vi "ITM10_test.vi"(7 "channel":i32=1, 11 "visa_in":refnum<visa-resource-name>="COM34") -> (0 "err_out":errorcluster={"status"=FALSE, "code"=1073676294, "source"="VISA Read in thcd_get_chan.vi"}, 2 "value":dbl, 4 "status":bool=TRUE, 5 "message":string)   [LabVIEW 2019]
panel:
  out "response V":string
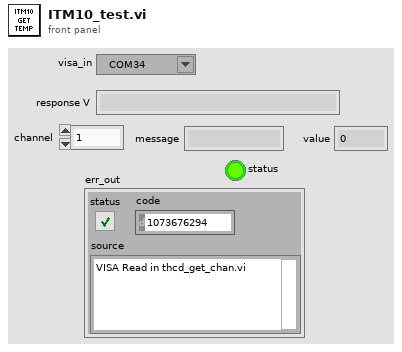
[diagram p1: front panel]
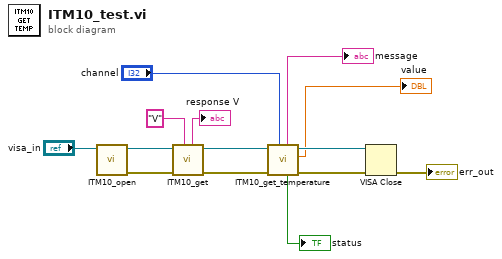
[diagram p0: block diagram]
diagram:
  n1 = call "ITM10_open.vi"("VISA in"="visa_in") -> ("error out"=w3:errorcluster, "VISA out"=w2:refnum<visa-resource-name>)  [unwired: 9 in]
  n2 = call "ITM10_get.vi"("command"="V", "error in"=w3, "VISA_ref_in"=w2) -> ("error out"=w10:errorcluster, "VISA_ref_out"=w11:refnum<visa-resource-name>, "response"=→"response V":string)  [unwired: 5 in, 1 out]
  n3 = call "ITM10_get_temperature.vi"("channel"="channel", "err_in"=w10, "visa_in"=w11) -> ("err_out"=w6:errorcluster, "temp"=→"value":dbl, "visa_out"=w7:refnum<visa-resource-name>, "status"=→"status":bool, "message"=→"message":string)  [unwired: 4 in]
  n4 = VISA Close(VISA resource name=w7, error in (no error)=w6) -> (error out=→"err_out":errorcluster)
